vi "Obtain Action Notifier.vi"(8 "error in (no error)":errorcluster) -> (0 "error out":errorcluster, 3 "notifier out":refnum<notifier>)   [LabVIEW 2014, in "Sprocket.lvlib"]
uses:
  Sprocket.lvlib
  src/Action/Action Name.ctl
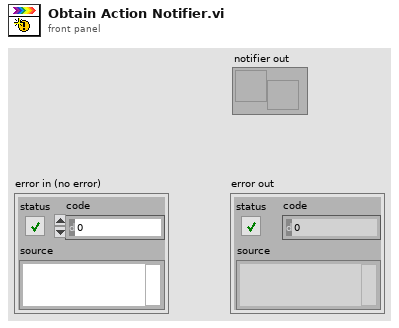
[diagram p1: front panel]
types:
  T1 = typedef "Sprocket.lvlib/Action Name.ctl" = enum16{"Drive Left", "Drive Right"}
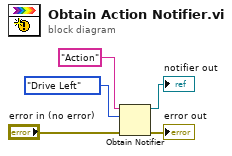
[diagram p0: block diagram]
diagram:
  n1 = Obtain Notifier(name (unnamed)="Action", notification data type=Action_Name."Drive Left" ("Name"), error in (no error)="error in (no error)") -> (notifier out=→"notifier out":refnum<notifier>, error out=→"error out":errorcluster)  [unwired: 1 in, 1 out]
